vi "Test Read Structs.vi"(11 "TwinCAT ADS in":refnum<class "TwinCAT ADS.lvclass">) -> (3 "TwinCAT ADS out":refnum<class "TwinCAT ADS.lvclass">)   [LabVIEW 2018]
uses:
  TwinCAT ADS Class/TwinCAT ADS.lvclass
  Controls/ST_Simple.ctl
  Controls/ST_Packed.ctl
  Controls/ST_Complex.ctl
  Controls/Enum.ctl
  Controls/FB_Simple.ctl
  0f192603-4b3d-4f37-814b-8045268a4184.vi
  67a72bd1-5191-48bf-9b9a-0a1df22764e4.vi
  c8f2f14a-791d-4484-b25b-25e31bed0e1d.vi
  0e82c4fa-873b-4361-ac99-2e6e4b7cd392.vi
  da0f88be-82f8-4e5b-86e7-5baa69d9b51e.vi
  4782b519-43e7-4b8e-bd72-e209be860882.vi
  e7a7b24b-aede-49d7-b369-bb451e1de87e.vi
  TwinCAT ADS Class/VIs/Data/Read.vi
  <vilib>/addons/_JKI Toolkits/Caraya/classes/Assert/Assert True.vi
  <vilib>/addons/_JKI Toolkits/Caraya/classes/Assert/Assert.lvclass
  <vilib>/addons/_JKI Toolkits/Caraya/classes/Test/Test.lvclass
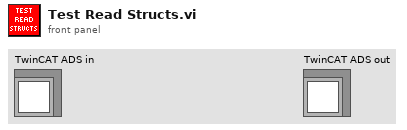
[diagram p1: front panel]
types:
  T1 = typedef "ST_Packed.ctl" = cluster{"bMember":bool, "dtMember":timestamp, "fMember":dbl}
  T2 = typedef "ST_Complex.ctl" = cluster{"bMember":bool, "eMember":T3, "stSimpleMember":T4, "stPackedMember":T1, "FB_Simple":T5, "arrfMember":dbl[]}
  T3 = typedef "Enum.ctl" = enum16{"Member 0", "Member 1", "Member 2"}
  T4 = typedef "ST_Simple.ctl" = cluster{"bMember":bool, "dtMember":timestamp, "nMember":i32}
  T5 = typedef "FB_Simple.ctl" = cluster{"_bMember":bool, "_nMember":i32, "_sMember":string}
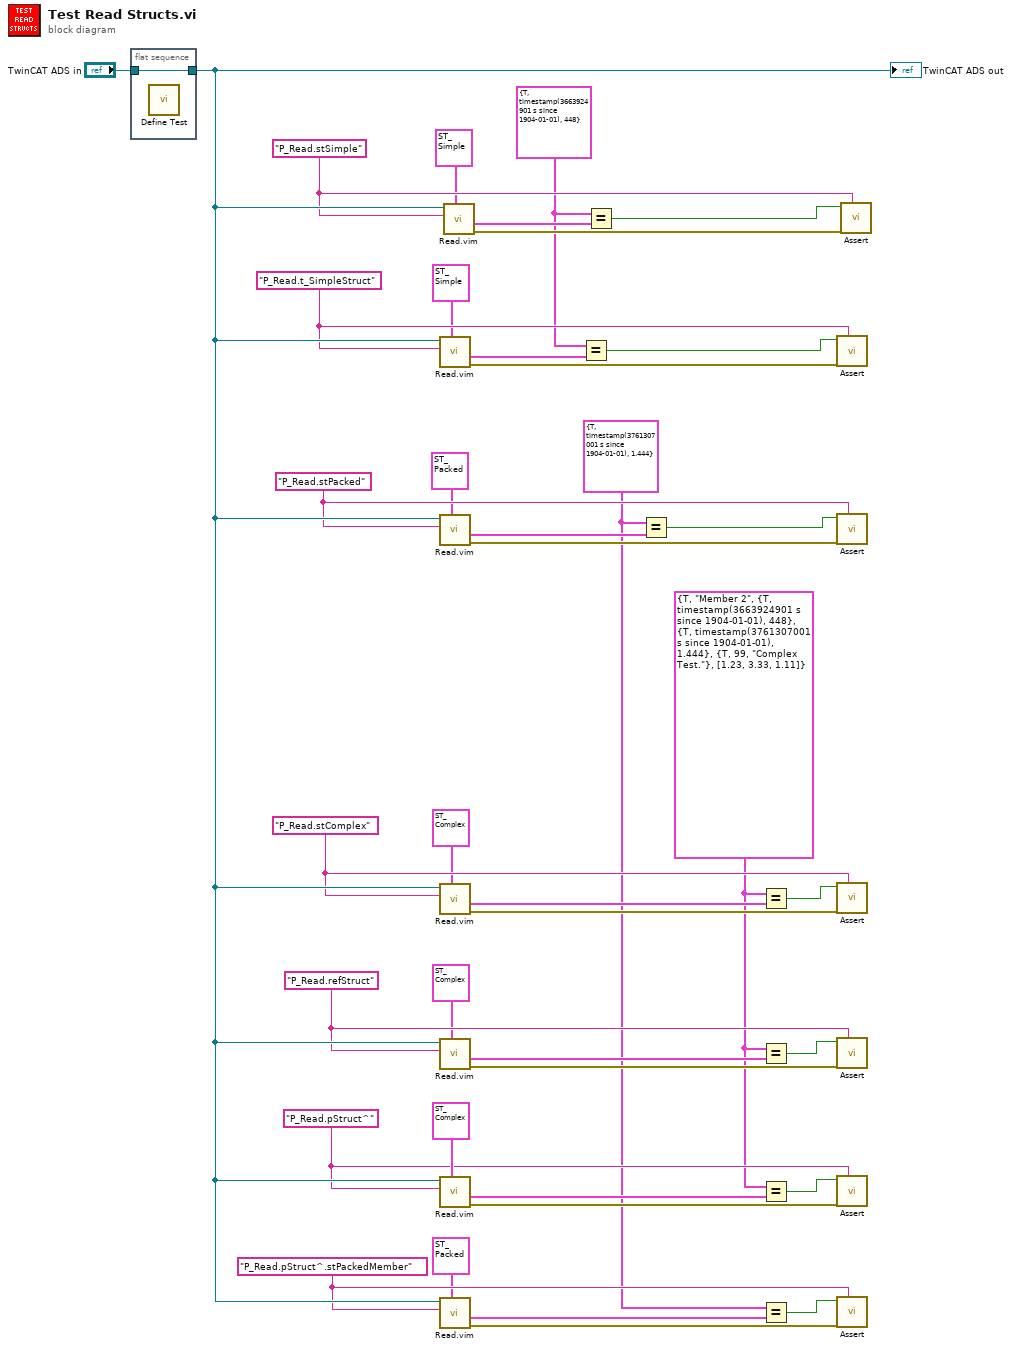
[diagram p0: block diagram]
diagram:
  w3 = "P_Read.pStruct^.stPackedMember" ("Symbol Name")
  w11 = "P_Read.pStruct^" ("Symbol Name")
  w14 = "P_Read.refStruct" ("Symbol Name")
  w7 = T2 {"bMember"=TRUE, "eMember"=enum."Member 2", "stSimpleMember"={"bMember"=TRUE, "dtMember"=timestamp(3663924901 s since 1904-01-01), "nMember"=448}, "stPackedMember"={"bMember"=TRUE, "dtMember"=timestamp(3761307001 s since 1904-01-01), "fMember"=1.444}, "FB_Simple"={"_bMember"=TRUE, "_nMember"=99, "_sMember"="Complex Test."}, "arrfMember"=[1.23, 3.33, 1.11]} ("ST_Complex")
  w1 = T1 {"bMember"=TRUE, "dtMember"=timestamp(3761307001 s since 1904-01-01), "fMember"=1.444} ("ST_Packed")
  w25 = T4 {"bMember"=TRUE, "dtMember"=timestamp(3663924901 s since 1904-01-01), "nMember"=448} ("ST_Simple")
  w32 = "P_Read.stComplex" ("Symbol Name")
  w33 = "P_Read.stPacked" ("Symbol Name")
  w36 = "P_Read.t_SimpleStruct" ("Symbol Name")
  w37 = "P_Read.stSimple" ("Symbol Name")
  n1 = flat-sequence {
    tunnel: "TwinCAT ADS in" -> [w41]
    tunnel: [w41] -> w40
    frame #0 {
      n2 = call <vilib>:"Define Test.vi"() -> ()  [unwired: 10 in, 2 out]
    }
  }
  n3 = call "Read.vim"("Type"=T4 {"bMember"=FALSE, "dtMember"=timestamp(0 s since 1904-01-01), "nMember"=0} ("ST_Simple"), "Symbol Name"=w36, "TwinCAT ADS in"=w40) -> ("error out"=w35:errorcluster, "Value"=w26:T4)  [unwired: 6 in, 1 out]
  n4 = call "Read.vim"("Type"=T1 {"bMember"=FALSE, "dtMember"=timestamp(0 s since 1904-01-01), "fMember"=0.0} ("ST_Packed"), "Symbol Name"=w33, "TwinCAT ADS in"=w40) -> ("error out"=w34:errorcluster, "Value"=w22:T1)  [unwired: 6 in, 1 out]
  n5 = call "Read.vim"("Type"=T2 {"bMember"=FALSE, "eMember"=enum."Member 0", "stSimpleMember"={"bMember"=FALSE, "dtMember"=timestamp(0 s since 1904-01-01), "nMember"=0}, "stPackedMember"={"bMember"=FALSE, "dtMember"=timestamp(0 s since 1904-01-01), "fMember"=0.0}, "FB_Simple"={"_bMember"=FALSE, "_nMember"=0, "_sMember"=""}, "arrfMember"=[]} ("ST_Complex"), "Symbol Name"=w32, "TwinCAT ADS in"=w40) -> ("error out"=w31:errorcluster, "Value"=w19:T2)  [unwired: 6 in, 1 out]
  n6 = call "Read.vim"("Type"=T2 {"bMember"=FALSE, "eMember"=enum."Member 0", "stSimpleMember"={"bMember"=FALSE, "dtMember"=timestamp(0 s since 1904-01-01), "nMember"=0}, "stPackedMember"={"bMember"=FALSE, "dtMember"=timestamp(0 s since 1904-01-01), "fMember"=0.0}, "FB_Simple"={"_bMember"=FALSE, "_nMember"=0, "_sMember"=""}, "arrfMember"=[]} ("ST_Complex"), "Symbol Name"=w14, "TwinCAT ADS in"=w40) -> ("error out"=w15:errorcluster, "Value"=w16:T2)  [unwired: 6 in, 1 out]
  n7 = call "Read.vim"("Type"=T2 {"bMember"=FALSE, "eMember"=enum."Member 0", "stSimpleMember"={"bMember"=FALSE, "dtMember"=timestamp(0 s since 1904-01-01), "nMember"=0}, "stPackedMember"={"bMember"=FALSE, "dtMember"=timestamp(0 s since 1904-01-01), "fMember"=0.0}, "FB_Simple"={"_bMember"=FALSE, "_nMember"=0, "_sMember"=""}, "arrfMember"=[]} ("ST_Complex"), "Symbol Name"=w11, "TwinCAT ADS in"=w40) -> ("error out"=w10:errorcluster, "Value"=w9:T2)  [unwired: 6 in, 1 out]
  n8 = call "Read.vim"("Type"=T1 {"bMember"=FALSE, "dtMember"=timestamp(0 s since 1904-01-01), "fMember"=0.0} ("ST_Packed"), "Symbol Name"=w3, "TwinCAT ADS in"=w40) -> ("error out"=w4:errorcluster, "Value"=w5:T1)  [unwired: 6 in, 1 out]
  n9 = call "Read.vim"("Type"=T4 {"bMember"=FALSE, "dtMember"=timestamp(0 s since 1904-01-01), "nMember"=0} ("ST_Simple"), "Symbol Name"=w37, "TwinCAT ADS in"=w40) -> ("error out"=w39:errorcluster, "Value"=w29:T4)  [unwired: 6 in, 1 out]
  n10 = Equal?(x=w25, y=w26) -> (x = y?=w24:bool)
  n11 = Equal?(x=w25, y=w29) -> (x = y?=w28:bool)
  n12 = Equal?(x=w1, y=w22) -> (x = y?=w21:bool)
  n13 = Equal?(x=w7, y=w19) -> (x = y?=w18:bool)
  n14 = Equal?(x=w7, y=w16) -> (x = y?=w17:bool)
  n15 = Equal?(x=w7, y=w9) -> (x = y?=w8:bool)
  n16 = Equal?(x=w1, y=w5) -> (x = y?=w6:bool)
  n17 = call-poly <vilib>:"Assert.vi"("Label"=w36, "error in (no error)"=w35, "True?"=w24) -> ()  [unwired: 7 in, 2 out]
  n18 = call-poly <vilib>:"Assert.vi"("Label"=w33, "error in (no error)"=w34, "True?"=w21) -> ()  [unwired: 7 in, 2 out]
  n19 = call-poly <vilib>:"Assert.vi"("Label"=w32, "error in (no error)"=w31, "True?"=w18) -> ()  [unwired: 7 in, 2 out]
  n20 = call-poly <vilib>:"Assert.vi"("Label"=w14, "error in (no error)"=w15, "True?"=w17) -> ()  [unwired: 7 in, 2 out]
  n21 = call-poly <vilib>:"Assert.vi"("Label"=w11, "error in (no error)"=w10, "True?"=w8) -> ()  [unwired: 7 in, 2 out]
  n22 = call-poly <vilib>:"Assert.vi"("Label"=w3, "error in (no error)"=w4, "True?"=w6) -> ()  [unwired: 7 in, 2 out]
  n23 = call-poly <vilib>:"Assert.vi"("Label"=w37, "error in (no error)"=w39, "True?"=w28) -> ()  [unwired: 7 in, 2 out]
  "TwinCAT ADS out" <- w40
